vi "MA-K3BarcodeReader_Read.vi"(8 "error in (no error)":errorcluster, 11 "VISA Reference":refnum<visa-resource-name>) -> (0 "error out":errorcluster, 2 "Result":cluster{"Read?":bool, "Data":string}, 3 "VISA Reference":refnum<visa-resource-name>)   [LabVIEW 2019]
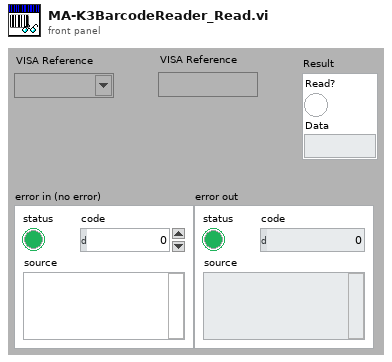
[diagram p1: front panel]
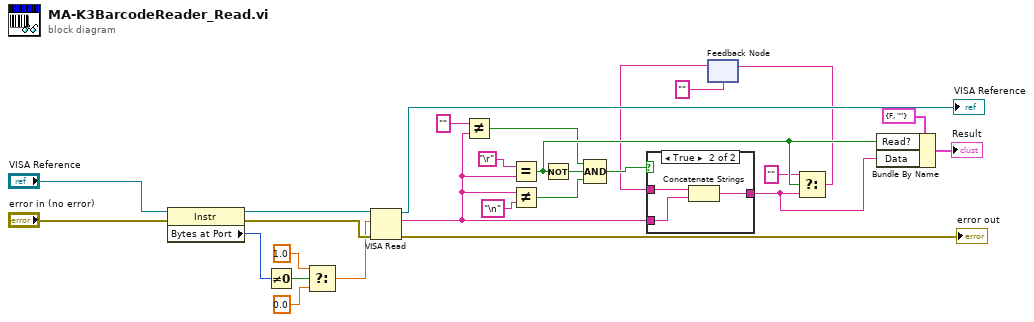
[diagram p0: block diagram]
diagram:
  n1 = property class="Instr"(reference="VISA Reference", error in="error in (no error)") -> (reference out=w19:refnum<visa-resource-name>, error out=w18:errorcluster, "Bytes at Port"=w15:u32)
  n2 = Not Equal To 0?(x=w15) -> (x != 0?=w14:bool)
  n3 = Select(t=1.0 ("f"), s=w14, f=0.0) -> (s? t:f=w16:dbl)
  n4 = VISA Read(VISA resource name=w19, byte count=w16, error in (no error)=w18) -> (VISA resource name out=→"VISA Reference":refnum<visa-resource-name>, read buffer=w3:string, error out=→"error out":errorcluster)  [unwired: 1 out]
  n5 = Not Equal?(x="" ("read buffer"), y=w3) -> (x != y?=w10:bool)
  n6 = Equal?(x="\r", y=w3) -> (x = y?=w23:bool)
  n7 = Not Equal?(x=w3, y="\n" ("read buffer")) -> (x != y?=w1:bool)
  n8 = Not(x=w23) -> (.not. x?=w8:bool)
  n9 = Compound Arithmetic op=AND(w10, w8, w1) -> (w9:bool)
  n10 = feedback #1("") -> (w6:string)
  n11 = case shown="True" w9 {
    tunnel: w3 -> [_ w31]
    tunnel: [w28 w30] -> w22
    tunnel: w6 -> [w28 w29]
    frame False {
    }
    frame True {
      n12 = Concatenate Strings(w29, w31) -> (w30:string)
    }
  }
  n13 = Select(t="", s=w23, f=w22) -> (s? t:f=w5:string)
  n14 = feedback-in #1(w5) -> ()
  n15 = Bundle By Name(cluster=cluster{"Read?":bool, "Data":string} {"Read?"=FALSE, "Data"=""} ("Result 2"), "Read?"=w23, "Data"=w22) -> (→"Result":cluster{"Read?":bool, "Data":string})
